vi "RunOperation.vi"(10 "Inputs":string[](array[string]), 11 "SaveForPrevious in":refnum<class "SaveForPrevious.lvclass">) -> (1 "Output/Failure":string, 2 "CLI Process Return Code":i32, 3 "SaveForPrevious out":refnum<class "SaveForPrevious.lvclass">)   [LabVIEW 2014, in "SaveForPrevious.lvclass"]
doc: "Entry point for LabVIEWCLI."
uses:
  SaveForPrevious.lvclass
  SaveForPrevious.lvclass/SaveForPrevious.ctl
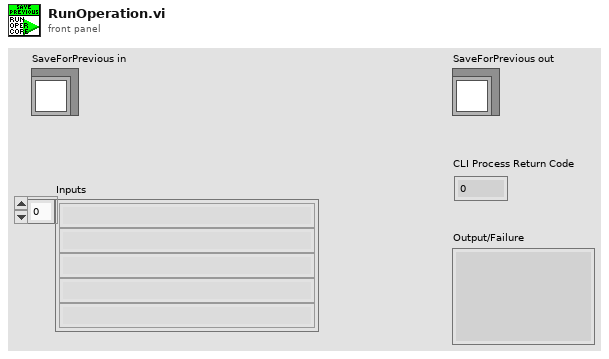
[diagram p1: front panel]
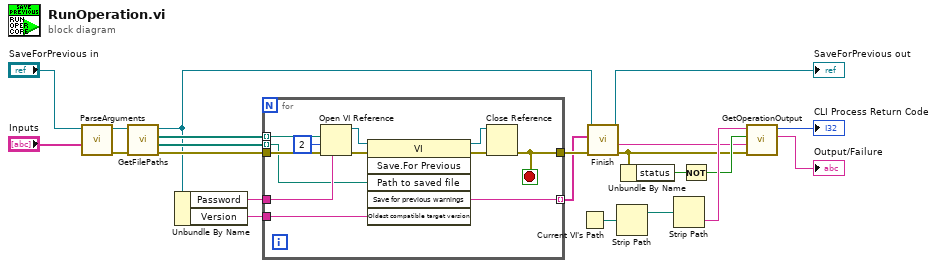
[diagram p0: block diagram]
diagram:
  n1 = call "ParseArguments.vi"("Inputs"="Inputs", "SaveForPrevious in"="SaveForPrevious in") -> ("error out"=w20:errorcluster, "SaveForPrevious out"=w8:refnum<class "SaveForPrevious.lvclass">)  [unwired: 8 in]
  n2 = call "GetFilePaths.vi"("error in (no error)"=w20, "SaveForPrevious in"=w8) -> ("error out"=w10:errorcluster, "Destinations"=w7:path[], "Sources"=w9:path[], "SaveForPrevious out"=w4:refnum<class "SaveForPrevious.lvclass">)  [unwired: 6 in]
  n3 = Unbundle By Name(w4) -> ("Password"=w19:string, "Version"=w18:string)
  n4 = for {
    tunnel: w10 -> [w34]
    tunnel: w9 -> [w28] mode=indexing
    tunnel: w19 -> [w31]
    tunnel: w18 -> [w30]
    tunnel: [w26] -> w6
    tunnel: w7 -> [w24] mode=indexing
    tunnel: [w23] -> w5 mode=indexing
    stop <- w26 stop-if-true
    n5 = Open VI Reference(vi path=w28, options=2, password ("")=w31, error in (no error)=w34) -> (vi reference=w29:refnum<vi>, error out=w33:errorcluster)  [unwired: 2 in]
    n6 = invoke class="VI" method="Save.For Previous"(reference=w29, error in=w33, "Path to saved file"=w24, "Oldest compatible target version"=w30) -> (reference out=w25:refnum<vi>, error out=w27:errorcluster, "Save for previous warnings"=w23:string)  [unwired: 2 in, 3 out]
    n7 = Close Reference(reference=w25, error in (no error)=w27) -> (error out=w26:errorcluster)
  }
  n8 = Current VI's Path() -> (path=w17:path)
  n9 = call "Finish.vi"("error in (no error)"=w6, "Warnings"=w5, "SaveForPrevious in"=w4) -> ("error out"=w2:errorcluster, "Output/Failure"=w1:string, "SaveForPrevious out"=→"SaveForPrevious out":refnum<class "SaveForPrevious.lvclass">)  [unwired: 6 in]
  n10 = Strip Path(path=w17) -> (stripped path=w16:path)  [unwired: 1 out]
  n11 = Unbundle By Name(w2) -> ("status"=w14:bool)
  n12 = Strip Path(path=w16) -> (name=w15:string)  [unwired: 1 out]
  n13 = Not(x=w14) -> (.not. x?=w13:bool)
  n14 = call <nishared>:"GetOperationOutput.vi"("error in (no error)"=w2, "Operation Output/Error In"=w1, "Operation succeeded?"=w13, "Operation Name"=w15) -> ("Operation Output/Error Out"=→"Output/Failure":string, "CLI Process Return Code"=→"CLI Process Return Code":i32)  [unwired: 6 in]
